vi "test Array Handle.vi"(8 "error in (no error)":errorcluster, 11 "TestCase in":refnum<class "Data Structure Tests.lvclass">) -> (0 "error out":errorcluster, 3 "TestCase out":refnum<class "Data Structure Tests.lvclass">)   [LabVIEW 2020, in "Data Structure Tests.lvclass"]
uses:
  Data Structure Tests.lvclass
  Data Structure Tests.lvclass/Data Structure Tests.ctl
  <vilib>/addons/_JKI Toolkits/VI Tester/TestCase.llb/TestCase.lvclass
  C:/Program Files (x86)/National Instruments/LabVIEW 2020/vi.lib/addons/_JKI Toolkits/VI Tester/TestCase.llb/TestCase.lvclass
panel:
  out "data string":string
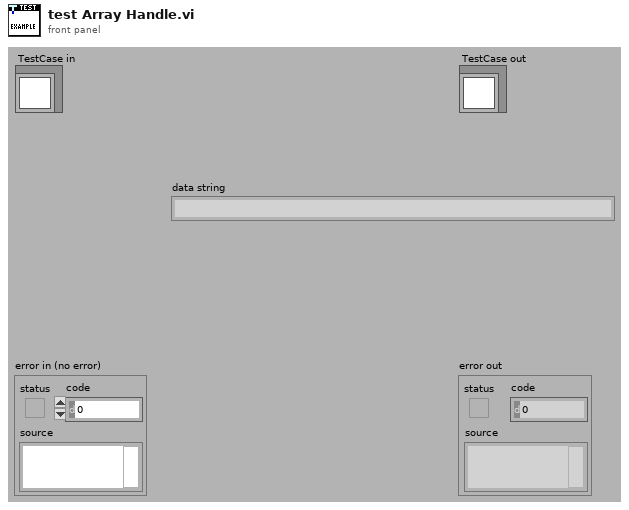
[diagram p1: front panel]
types:
  T1 = enum16{"big-endian, network order", "native, host order", "little-endian"}
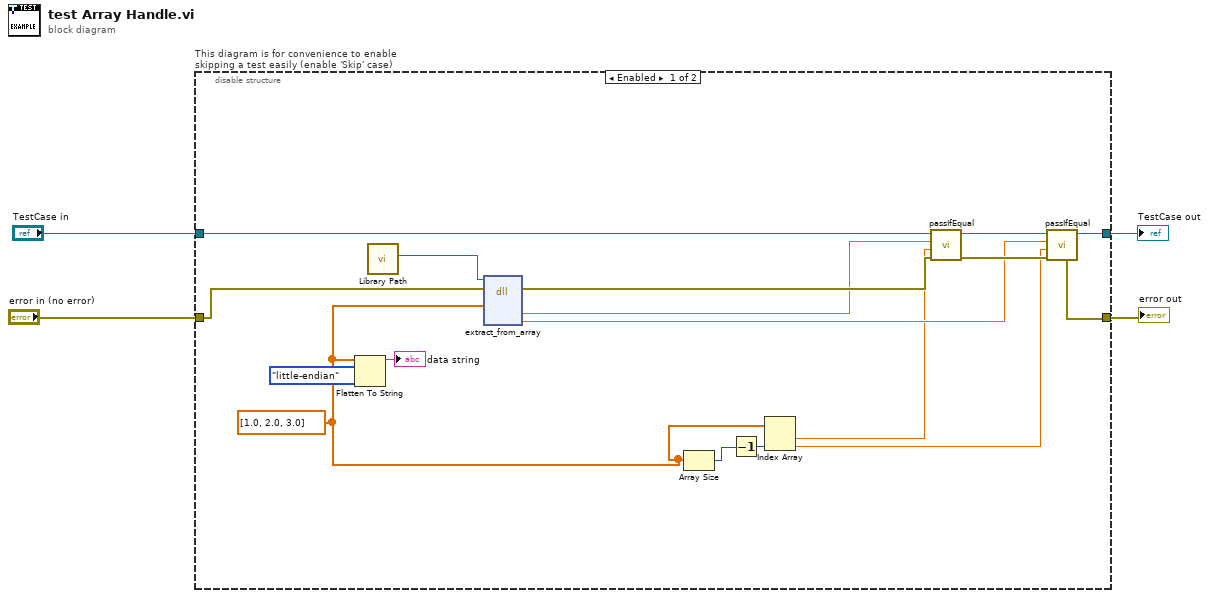
[diagram p0: block diagram]
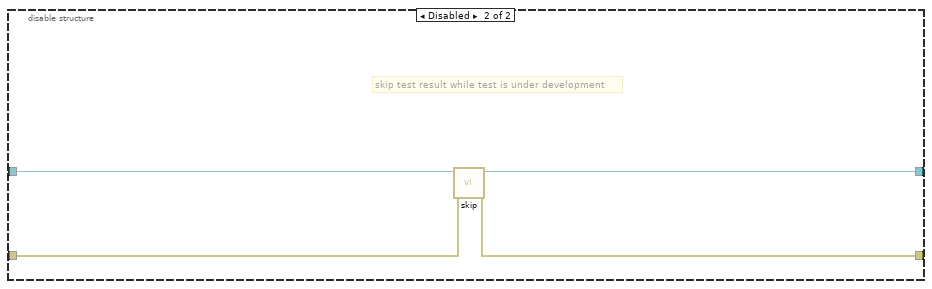
[diagram p2: hidden frame]
diagram:
  n1 = disable-structure "This diagram is for convenience to enable skipping a test easily (enable 'Skip' case)" shown="Enabled" {
    disable-tunnel: "TestCase in" -> [w21 w25]
    disable-tunnel: [w15 w23] -> w1
    disable-tunnel: [w17 w24] -> w3
    disable-tunnel: "error in (no error)" -> [w20 w22]
    frame Enabled {
      w7 = dbl[] [1.0, 2.0, 3.0] ("Y")
      n2 = Flatten To String(anything=w7, byte order (0:big-endian, network order)=T1."little-endian") -> (data string=→"data string":string)  [unwired: 2 in, 2 out]
      n3 = call "Library Path.vi"() -> ("Library Path"=w8:path)  [unwired: 11 in]
      n4 = dll-call lib="C:/Users/JamesMcNally/Documents/RustInterop/Rust-LabVIEW-Interop/target/debug/labview_test_library.dll" fn="extract_from_array"(path in=w8, error in=w20, "array"=w7) -> (error out=w19:errorcluster, "wv_first"=w14:dbl, "wv_last"=w13:dbl)  [unwired: 5 in, 1 out]
      n5 = Array Size(array=w7) -> (size(s)=w11:i32)
      n6 = Decrement(x=w11) -> (x-1=w10:i32)
      n7 = Index Array(array=w7, index #2=w10) -> (element #1=w12:dbl, element #2=w9:dbl)  [unwired: 1 in]
      n8 = call-dynamic "passIfEqual.vi"("error in (no error)"=w19, "y"=w12, "x"=w14, "TestCase in"=w21) -> ("error out"=w18:errorcluster, "TestCase out"=w16:refnum<class "Data Structure Tests.lvclass">)  [unwired: 6 in]
      n9 = call-dynamic "passIfEqual.vi"("error in (no error)"=w18, "y"=w9, "x"=w13, "TestCase in"=w16) -> ("error out"=w17:errorcluster, "TestCase out"=w15:refnum<class "Data Structure Tests.lvclass">)  [unwired: 6 in]
    }
    frame Disabled {
      # "skip test result while test is under development"
      n10 = call <vilib>:"skip.vi"("error in (no error)"=w22, "TestCase in"=w25) -> ("error out"=w24:errorcluster, "TestCase out"=w23:refnum<class "Data Structure Tests.lvclass">)  [unwired: 8 in]
    }
  }
  "error out" <- w3
  "TestCase out" <- w1
